vi "Immediate Children.vi"(8 "error in":errorcluster, 9 "Type File Path":path, 10 "Project:Active Project":refnum<vi>) -> (0 "error out":errorcluster, 2 "Implemented Class File Paths":path[](array[path]))   [LabVIEW 2025, in "_Shared.lvlib"]
uses:
  _Shared.lvlib
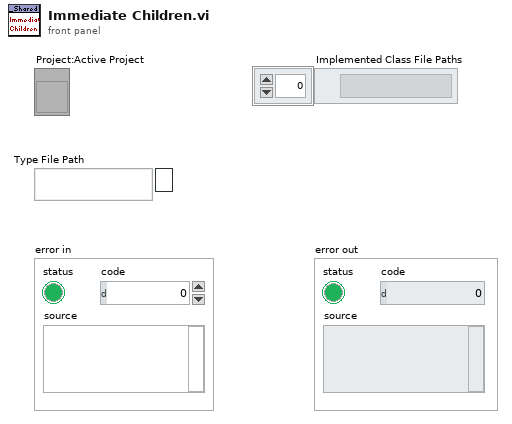
[diagram p1: front panel]
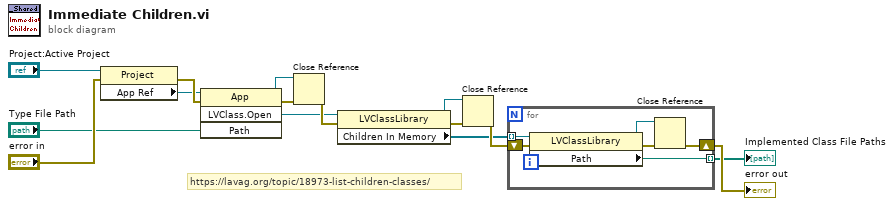
[diagram p0: block diagram]
diagram:
  # "https://lavag.org/topic/18973-list-children-classes/"
  n1 = property class="Project"(reference="Project:Active Project", error in="error in") -> (error out=w4:errorcluster, "App Ref"=w1:refnum<vi>)  [unwired: 1 out]
  n2 = invoke class="App" method="LVClass.Open"(reference=w1, error in=w4, "Path"="Type File Path") -> (reference out=w15:refnum<vi>, error out=w14:errorcluster, "LVClass.Open"=w12:refnum<vi>)  [unwired: 1 in, 1 out]
  n3 = Close Reference(reference=w15, error in (no error)=w14) -> (error out=w13:errorcluster)
  n4 = property class="LVClassLibrary"(reference=w12, error in=w13) -> (reference out=w10:refnum<vi>, error out=w11:errorcluster, "Children In Memory"=w8:refnum<vi>[])
  n5 = Close Reference(reference=w10, error in (no error)=w11) -> (error out=w9:errorcluster)
  n6 = for {
    tunnel: w8 -> [w20] mode=indexing
    shift-right: [w17] -> w7
    shift-left: w9 -> [w21]
    tunnel: [w16] -> w6 mode=indexing
    n7 = property class="LVClassLibrary"(reference=w20, error in=w21) -> (reference out=w18:refnum<vi>, error out=w19:errorcluster, "Path"=w16:path)
    n8 = Close Reference(reference=w18, error in (no error)=w19) -> (error out=w17:errorcluster)
  }
  "error out" <- w7
  "Implemented Class File Paths" <- w6
